vi "Zamena (SubVI).vi"(8 "comm?":bool, 11 "input string":string) -> (3 "result string 2":string)   [LabVIEW 2017]
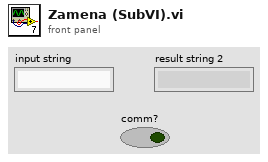
[diagram p1: front panel]
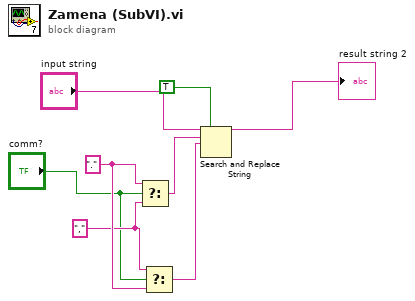
[diagram p0: block diagram]
diagram:
  w4 = ","
  w5 = "."
  n1 = Select(t=w5, s="comm?", f=w4) -> (s? t:f=w6:string)
  n2 = Select(t=w4, s="comm?", f=w5) -> (s? t:f=w3:string)
  n3 = Search and Replace String(replace all?=TRUE ("replace all? (F)"), input string="input string", search string=w6, replace string=w3) -> (result string=→"result string 2":string)  [unwired: 4 in, 3 out]
